vi "Configure Event Search (Glitch).vi"(5 "High Limit (3E-9 S)":dbl=3e-09, 6 "Low Limit (2E-9 S)":dbl=2e-09, 7 "Polarity (0: Positive)":i32(ring) items=["Positive", "Negative"], 8 "error in (no error)":errorcluster, 9 "Qualifier (1: Less Than)":i32(ring)=1 items=["Greater Than", "Less Than", "Range"], 10 "Source Channel (0: Channel 1)":i32(ring) items=["Channel 1", "Channel 2", "Channel 3", "Channel 4"], 11 "VISA resource name":refnum<visa-resource-name>) -> (0 "error out":errorcluster, 3 "VISA resource name out":refnum<visa-resource-name>)   [LabVIEW 2023, in "Keysight-DSQx3014T.lvlib"]
doc: "Configures the event search of Glitch."
uses:
  Keysight-DSQx3014T.lvlib
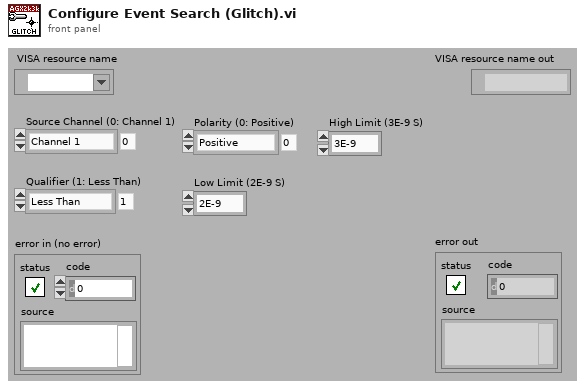
[diagram p1: front panel]
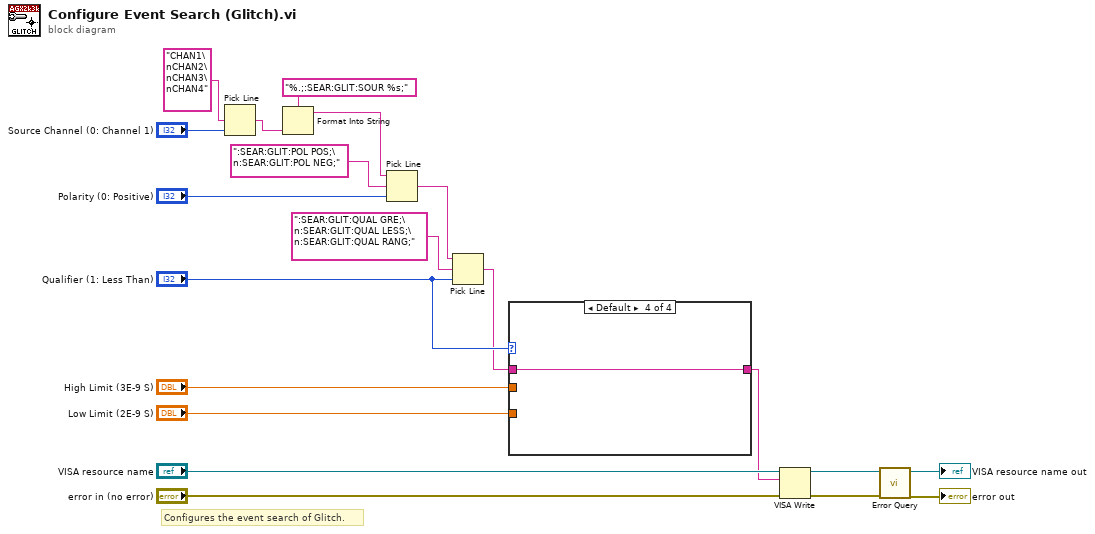
[diagram p0: block diagram]
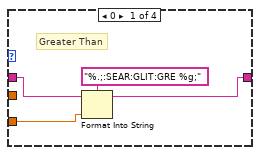
[diagram p2: hidden frame]
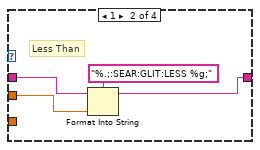
[diagram p3: hidden frame]
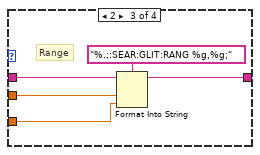
[diagram p4: hidden frame]
diagram:
  # "Configures the event search of Glitch."
  n1 = Pick Line(multi-line string="CHAN1\nCHAN2\nCHAN3\nCHAN4", line index="Source Channel (0: Channel 1)") -> (output string=w1:string)  [unwired: 1 out]
  n2 = Format Into String(format string="%.;:SEAR:GLIT:SOUR %s;", w1) -> (resulting string=w9:string)  [unwired: 2 in, 1 out]
  n3 = Pick Line(string ("")=w9, multi-line string=":SEAR:GLIT:POL POS;\n:SEAR:GLIT:POL NEG;", line index="Polarity (0: Positive)") -> (output string=w17:string)
  n4 = Pick Line(string ("")=w17, multi-line string=":SEAR:GLIT:QUAL GRE;\n:SEAR:GLIT:QUAL LESS;\n:SEAR:GLIT:QUAL RANG;", line index="Qualifier (1: Less Than)") -> (output string=w5:string)
  n5 = case shown="Default" "Qualifier (1: Less Than)" {
    tunnel: "High Limit (3E-9 S)" -> [_ w27 w32 _]
    tunnel: "Low Limit (2E-9 S)" -> [w23 _ w31 _]
    tunnel: w5 -> [w21 w26 w30 w34]
    tunnel: [w22 w25 w29 w34] -> w4
    frame 0 {
      # "Greater Than"
      n6 = Format Into String(format string="%.;:SEAR:GLIT:GRE %g;", initial string=w21, w23) -> (resulting string=w22:string)  [unwired: 1 in, 1 out]
    }
    frame 1 {
      # "Less Than"
      n7 = Format Into String(format string="%.;:SEAR:GLIT:LESS %g;", initial string=w26, w27) -> (resulting string=w25:string)  [unwired: 1 in, 1 out]
    }
    frame 2 {
      # "Range"
      n8 = Format Into String(format string="%.;:SEAR:GLIT:RANG %g,%g;", initial string=w30, w32, w31) -> (resulting string=w29:string)  [unwired: 1 in, 1 out]
    }
    frame Default {
    }
  }
  n9 = VISA Write(VISA resource name="VISA resource name", write buffer=w4, error in (no error)="error in (no error)") -> (VISA resource name out=w14:refnum<visa-resource-name>, error out=w13:errorcluster)  [unwired: 1 out]
  n10 = call "Error Query.vi"("error in (no error)"=w13, "VISA resource name"=w14) -> ("error out"=→"error out":errorcluster, "VISA resource name out"=→"VISA resource name out":refnum<visa-resource-name>)  [unwired: 8 out]
